vi "CompareLastHWI_DDS.vi"(9 "Last DDS HWI cluster":T1={"Device Identifiers"={"Channel Name"="", "Handle"=-1}, "Device Settings"={"Sweeps"=FALSE, "PB trig / Sequence"=FALSE, "Amp Lock"=FALSE, "Firmware Ver"=0.0}, "Hardware Image"={"Freq. 0 [MHz]"=[], "Freq. 1 [MHz]"=[], "Amp [Level]"=[], "Phase  [deg]"=[], "Swp Dir [0/1]"=[], "Swp Time [sec]"=[]}}, 10 "DDS HWI cluster":T1={"Device Identifiers"={"Channel Name"="", "Handle"=-1}, "Device Settings"={"Sweeps"=FALSE, "PB trig / Sequence"=FALSE, "Amp Lock"=FALSE, "Firmware Ver"=0.0}, "Hardware Image"={"Freq. 0 [MHz]"=[], "Freq. 1 [MHz]"=[], "Amp [Level]"=[], "Phase  [deg]"=[], "Swp Dir [0/1]"=[], "Swp Time [sec]"=[]}}) -> (2 "change?":bool)   [LabVIEW 2013]
doc: "Compare next to last DDS hardware info (Device identifiers, Device settings, and Hardware Image). Output \"change?\" boolean if ANYTHING changes."
uses:
  Utils/Unequal_safe/Unequal_Safe_1dDBL.vi
  Utils/Unequal_safe/Unequal_Safe_1dI32.vi
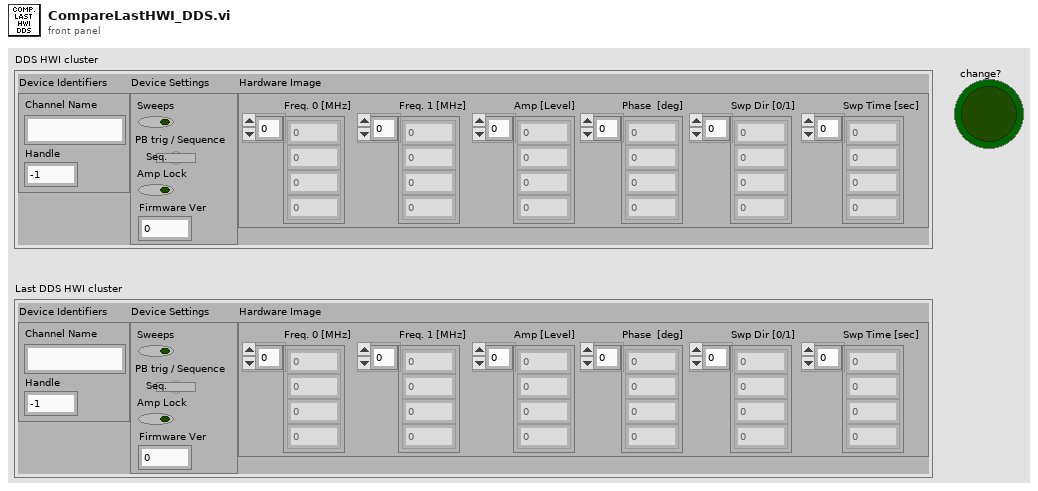
[diagram p1: front panel]
types:
  T1 = cluster{"Device Identifiers":cluster{"Channel Name":string, "Handle":i64}, "Device Settings":cluster{"Sweeps":bool, "PB trig / Sequence":bool, "Amp Lock":bool, "Firmware Ver":dbl}, "Hardware Image":cluster{"Freq. 0 [MHz]":dbl[], "Freq. 1 [MHz]":dbl[], "Amp [Level]":dbl[], "Phase  [deg]":dbl[], "Swp Dir [0/1]":i32[], "Swp Time [sec]":dbl[]}}
  T2 = cluster{"Sweeps":bool, "PB trig / Sequence":bool, "Amp Lock":bool, "Firmware Ver":dbl}
  T3 = cluster{"Sweeps":bool, "PB trig / Sequence":bool, "Amp Lock":bool, "Firmware Ver":bool}
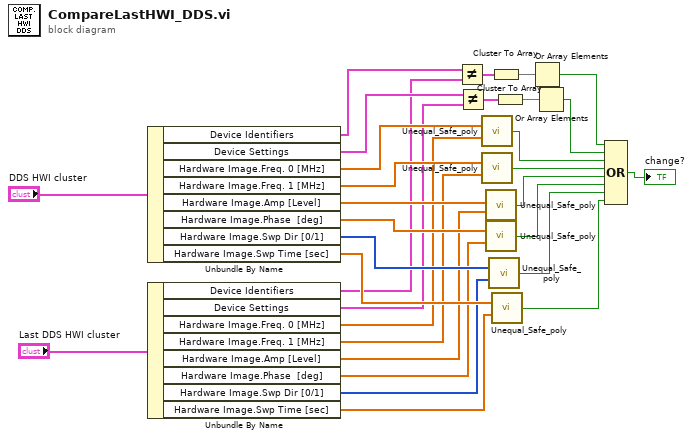
[diagram p0: block diagram]
diagram:
  n1 = Unbundle By Name("DDS HWI cluster") -> ("Device Identifiers"=w29:cluster{"Channel Name":string, "Handle":i64}, "Device Settings"=w28:T2, "Hardware Image.Freq. 0 [MHz]"=w27:dbl[], "Hardware Image.Freq. 1 [MHz]"=w26:dbl[], "Hardware Image.Amp [Level]"=w25:dbl[], "Hardware Image.Phase  [deg]"=w24:dbl[], "Hardware Image.Swp Dir [0/1]"=w23:i32[], "Hardware Image.Swp Time [sec]"=w22:dbl[])
  n2 = Unbundle By Name("Last DDS HWI cluster") -> ("Device Identifiers"=w8:cluster{"Channel Name":string, "Handle":i64}, "Device Settings"=w5:T2, "Hardware Image.Freq. 0 [MHz]"=w4:dbl[], "Hardware Image.Freq. 1 [MHz]"=w3:dbl[], "Hardware Image.Amp [Level]"=w2:dbl[], "Hardware Image.Phase  [deg]"=w1:dbl[], "Hardware Image.Swp Dir [0/1]"=w6:i32[], "Hardware Image.Swp Time [sec]"=w7:dbl[])
  n3 = Not Equal?(x=w29, y=w8) -> (x != y?=w21:cluster{"Channel Name":bool, "Handle":bool})
  n4 = Not Equal?(x=w28, y=w5) -> (x != y?=w18:T3)
  n5 = call-poly "Unequal_Safe_poly.vi"("x"=w27, "y"=w4) -> ("Diff?"=w15:bool)  [unwired: 12 in, 1 out]
  n6 = call-poly "Unequal_Safe_poly.vi"("x"=w26, "y"=w3) -> ("Diff?"=w14:bool)  [unwired: 12 in, 1 out]
  n7 = call-poly "Unequal_Safe_poly.vi"("x"=w25, "y"=w2) -> ("Diff?"=w13:bool)  [unwired: 12 in, 1 out]
  n8 = call-poly "Unequal_Safe_poly.vi"("x"=w24, "y"=w1) -> ("Diff?"=w12:bool)  [unwired: 12 in, 1 out]
  n9 = call-poly "Unequal_Safe_poly.vi"("x"=w23, "y"=w6) -> ("Diff?"=w11:bool)  [unwired: 12 in, 1 out]
  n10 = Cluster To Array(cluster=w21) -> (array=w20:bool[])
  n11 = call-poly "Unequal_Safe_poly.vi"("x"=w22, "y"=w7) -> ("Diff?"=w10:bool)  [unwired: 12 in, 1 out]
  n12 = Cluster To Array(cluster=w18) -> (array=w19:bool[])
  n13 = Or Array Elements(Boolean array=w20) -> (logical OR=w17:bool)
  n14 = Or Array Elements(Boolean array=w19) -> (logical OR=w16:bool)
  n15 = Compound Arithmetic op=OR(w17, w16, w15, w14, w13, w12, w11, w10) -> (→"change?":bool)
